vi "Main.vi"(11 "Module Admin":refnum<class "Delacor_lib_QMH_Module Admin.lvclass">) -> ()   [LabVIEW 2020, in "Numpad.lvlib"]
doc: "This template is based off of the Queued Message Handler design pattern and the Queued Message Handler project template that ships with LabVIEW.\n\nThe main difference is that the queue is private to this module and communication between modules is performed via Broadcast and Request events.\n\nRequest events are wrapped in public API methods and are handled in the Event Handling Loop (EHL) of this VI. Any module can register for Broadcast events sent by this module. The EHL generates messages based on user interface actions.\n\nThe Message Handling Loop (MHL) processes messages generated by the EHL, or by other messages. The messages are string values, so new messages can be added easily to the Message Cases case structure in the MHL. Each message cluster can also provide an optional value for Message Data, which is a variant that can be converted to whatever message-specific data is required.\n_____\nBased on Delacor QMH Project Template 5.0.0.82."
uses:
  Numpad.lvlib
  <vilib>/Delacor/Delacor QMH/Libraries/Module Admin_class/Delacor_lib_QMH_Module Admin.lvclass
  Module Data--cluster.ctl
  Stop Argument--cluster.ctl
  <vilib>/Delacor/Delacor QMH/Libraries/Message Queue_class/Delacor_lib_QMH_Message Queue.lvclass/Delacor_lib_QMH_Message Queue.ctl
  <vilib>/Delacor/Delacor QMH/Libraries/Module Admin_class/Delacor_lib_QMH_Module Admin.lvclass/Delacor_lib_QMH_Module Admin.ctl
  Insertar en Subpanel Argument--cluster.ctl
  <vilib>/Utility/miscctls.llb/LVPointTypeDef.ctl
  <vilib>/Delacor/Delacor QMH/Libraries/Message Queue_class/Delacor_lib_QMH_Enqueue Message (Single).vi
  <vilib>/Delacor/Delacor QMH/Libraries/Module Admin_class/Delacor_lib_QMH_Get External Launch.vi
  <vilib>/Utility/error.llb/Error Cluster From Error Code.vi
  <vilib>/ErrorRing/Error Ring.xnode
  <vilib>/Delacor/Delacor QMH/Libraries/Message Queue_class/Delacor_lib_QMH_Message Queue.lvclass
panel:
  out "number":i32
  in  "ok":bool
  in  "0":bool
  in  "del":bool
  in  "9":bool
  in  "8":bool
  in  "7":bool
  in  "6":bool
  in  "5":bool
  in  "4":bool
  in  "3":bool
  in  "2":bool
  in  "1":bool
  out "error out":errorcluster
  out "Status":string
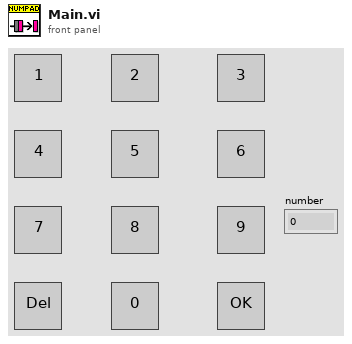
[diagram p1: front panel]
types:
  T1 = typedef "Numpad.lvlib/Request Events--cluster.ctl" = cluster{"Stop Module":refnum<user-event>, "Show Panel":refnum<user-event>, "Hide Panel":refnum<user-event>, "Get Module Execution Status":refnum<user-event>, "Show Diagram":refnum<user-event>, "Insertar en Subpanel":refnum<user-event>}
  T2 = typedef "Numpad.lvlib/Module Data--cluster.ctl" = cluster{"Status":string}
  T3 = enum32{"invalid lock state", "Not Locked", "Locked (No Password)", "Password-protected"}
  T4 = typedef "Numpad.lvlib/Stop Argument--cluster.ctl" = cluster{"Origin":string, "Exit via Stop Module Req?":bool, "Wait for Module to stop?":bool}
  T5 = typedef "Numpad.lvlib/Insertar en Subpanel Argument--cluster.ctl" = cluster{"Subpanel Ref":refnum<vi>}
  T6 = typedef "LVPointTypeDef.ctl" = cluster{"Horizontal":i16, "Vertical":i16}
  T7 = enum32{"Invalid", "Standard", "Closed", "Hidden", "Minimized", "Maximized"}
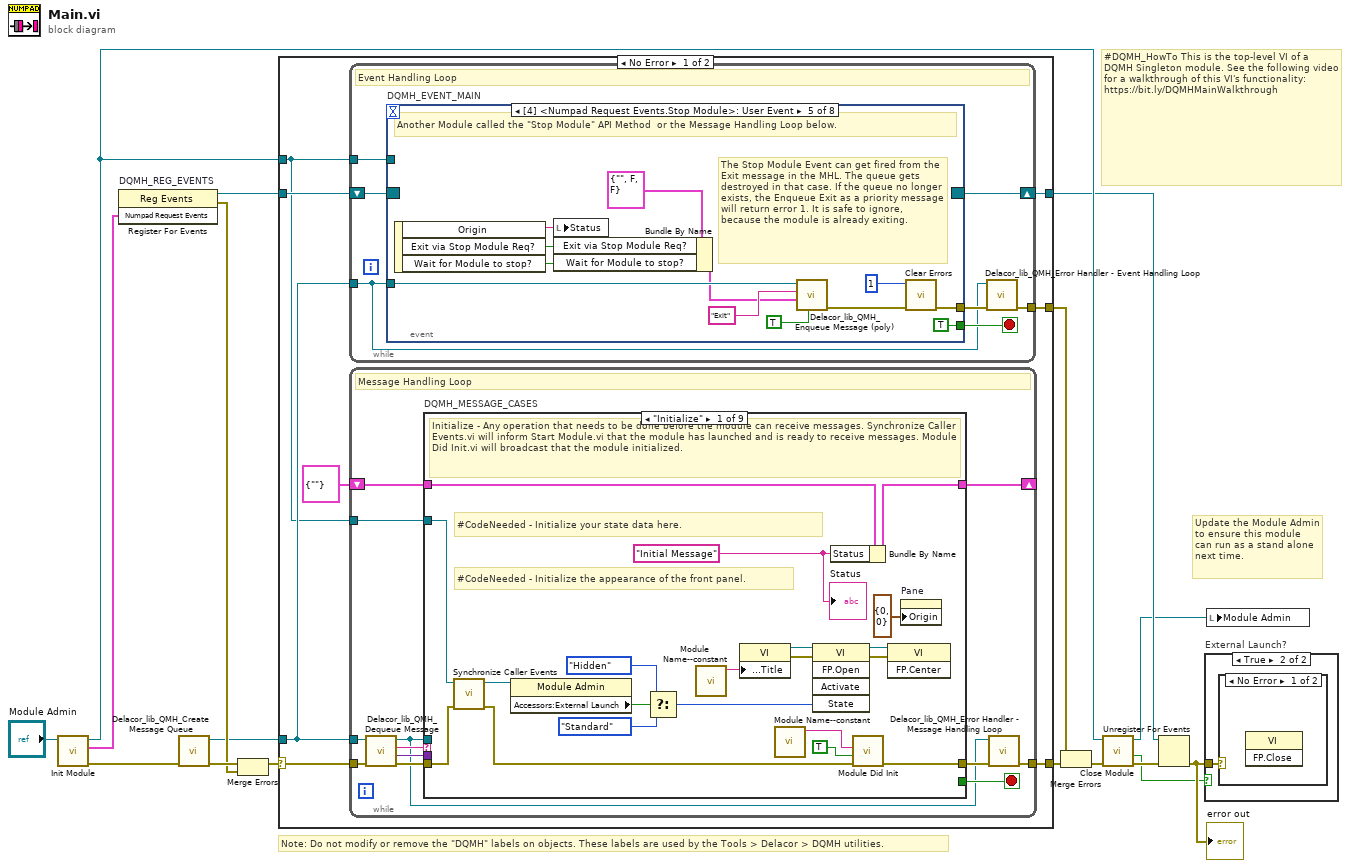
[diagram p0: block diagram]
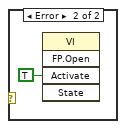
[diagram p3: hidden frame]
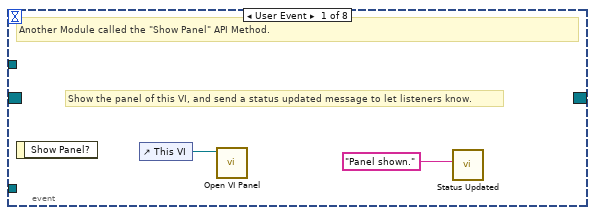
[diagram p4: hidden frame]
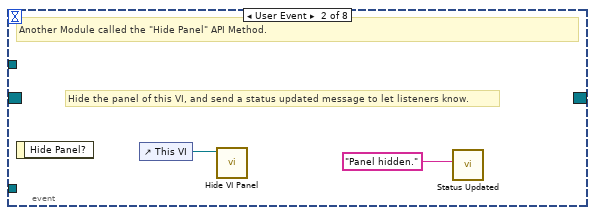
[diagram p5: hidden frame]
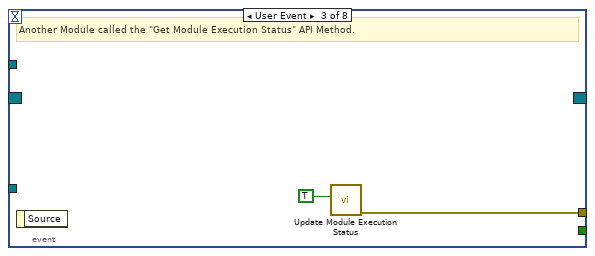
[diagram p6: hidden frame]
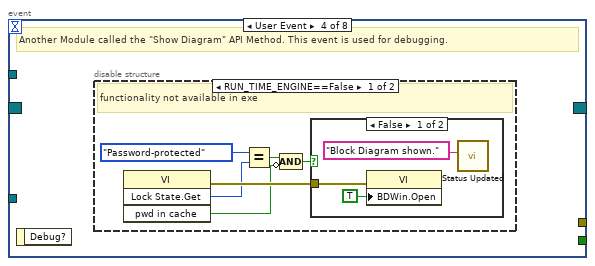
[diagram p7: hidden frame]
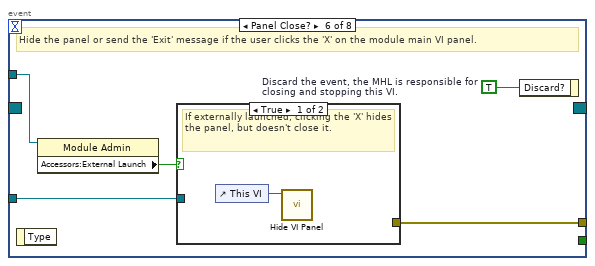
[diagram p10: hidden frame]
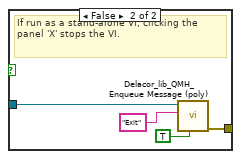
[diagram p11: hidden frame]
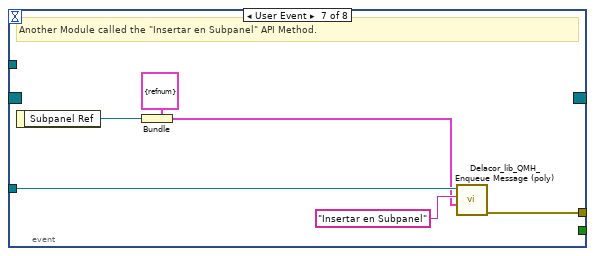
[diagram p12: hidden frame]
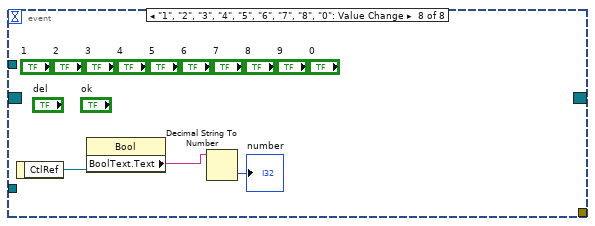
[diagram p13: hidden frame]
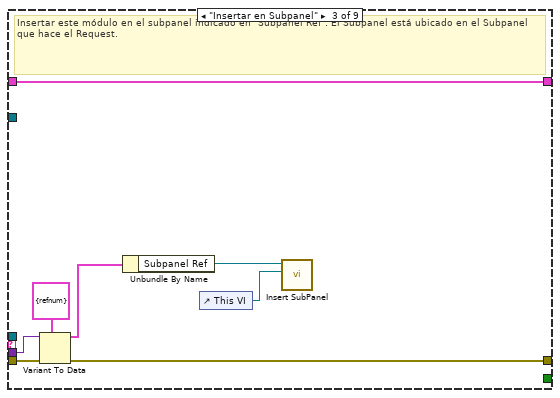
[diagram p15: hidden frame]
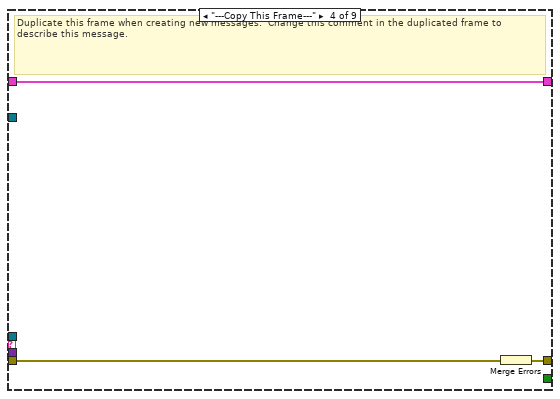
[diagram p16: hidden frame]
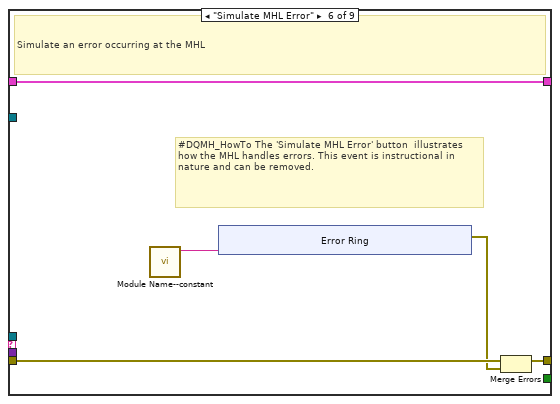
[diagram p18: hidden frame]
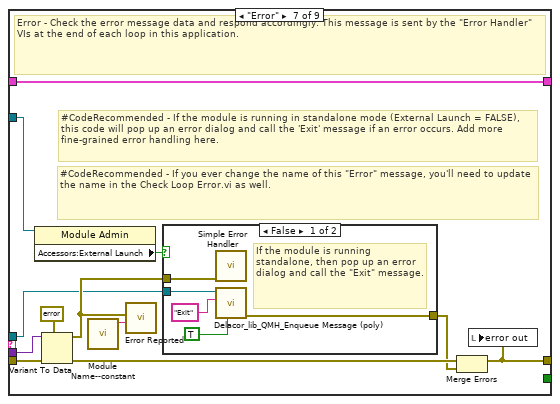
[diagram p19: hidden frame]
diagram:
  # "#DQMH_HowTo This is the top-level VI of a DQMH Singleton module. See the following video for a walkthrough of this VI's functionality: https://bit.ly/DQMHMainWalkthrough"
  # "Note: Do not modify or remove the \"DQMH\" labels on objects. These labels are used by the Tools > Delacor > DQMH utilities."
  # "Update the Module Admin to ensure this module can run as a stand alone next time."
  n1 = call "Init Module.vi"("Singleton Module Admin in"="Module Admin") -> ("error out"=w16:errorcluster, "Numpad Request Events"=w5:T1, "Singleton Module Admin out"=w8:refnum<class "Delacor_lib_QMH_Module Admin.lvclass">)  [unwired: 8 in]
  n2 = register-events "DQMH_REG_EVENTS"(w5) -> (reference out=w6:refnum<event-registration>, error out=w9:errorcluster)  [unwired: 2 in]
  n3 = call <vilib>:"Delacor_lib_QMH_Create Message Queue.vi"("error in (no error)"=w16) -> ("error out"=w11:errorcluster, "Message Queue"=w4:refnum<class "Delacor_lib_QMH_Message Queue.lvclass">)  [unwired: 9 in]
  n4 = Merge Errors(w11, w9) -> (w10:errorcluster)
  n5 = case shown="No Error" w10 {
    selector: w10 -> [w23 w186]
    tunnel: [w25 w185] -> w17
    tunnel: [w22 w191] -> w7
    tunnel: w6 -> [w20 w191]
    tunnel: w4 -> [w19 w184]
    tunnel: [w24 _] -> w14
    tunnel: w8 -> [w18 w187]
    frame No Error {
      n6 = while {
        tunnel: w19 -> [w26]
        shift-right: [w29] -> w22
        shift-left: w20 -> [w30]
        tunnel: [w31] -> w24
        tunnel: w18 -> [w27]
        stop <- w28 stop-if-true
        # "Event Handling Loop"
        n7 = event "DQMH_EVENT_MAIN" shown="[4] <Numpad Request Events.Stop Module>: User Event" {
          selector: w30 -> [_ _ _ _ _ _ _ _]
          dyn-events: [_ _ _ _ _ _ _ _] -> w29
          timeout: _ -> [_ _ _ _ _ _ _ _]
          tunnel: [_ _ _ _ TRUE ("Discard?") _ _ _] -> w28
          tunnel: w26 -> [_ _ _ _ w55 w62 w75 _]
          tunnel: [_ _ w38 _ w58 w64 w70 _] -> w32
          tunnel: w27 -> [_ _ _ _ _ w61 _ _]
          event User Event {
            # "Show the panel of this VI, and send a status updated message to let listeners know."
            # "Another Module called the \"Show Panel\" API Method."
            n8 = event-data() -> ()  [unwired: 1 in, 1 out]
            n9 = control-ref of="This VI"() -> (w34:refnum<vi>)
            n10 = call "Open VI Panel.vi"("VI"=w34) -> ()  [unwired: 10 in, 1 out]
            n11 = call "Status Updated.vi"("Status"="Panel shown." ("format string")) -> ()  [unwired: 10 in, 1 out]
          }
          event User Event {
            # "Hide the panel of this VI, and send a status updated message to let listeners know."
            # "Another Module called the \"Hide Panel\" API Method."
            n12 = event-data() -> ()  [unwired: 1 in, 1 out]
            n13 = control-ref of="This VI"() -> (w36:refnum<vi>)
            n14 = call "Hide VI Panel.vi"("VI"=w36) -> ()  [unwired: 10 in, 1 out]
            n15 = call "Status Updated.vi"("Status"="Panel hidden." ("format string")) -> ()  [unwired: 10 in, 1 out]
          }
          event User Event {
            # "Another Module called the \"Get Module Execution Status\" API Method."
            n16 = event-data() -> ()  [unwired: 1 in, 1 out]
            n17 = call "Update Module Execution Status.vi"("Running?"=TRUE) -> ("error out"=w38:errorcluster)  [unwired: 10 in]
          }
          event User Event {
            # "Another Module called the \"Show Diagram\" API Method. This event is used for debugging."
            n18 = event-data() -> ()  [unwired: 1 in, 1 out]
            n19 = disable-structure shown="RUN_TIME_ENGINE==False" {
              frame condition #0 (active) {
                # "functionality not available in exe"
                n20 = invoke class="VI" method="Lock State.Get"() -> (error out=w44:errorcluster, "Get Lock State"=w43:T3, "pwd in cache"=w40:bool)  [unwired: 4 in, 1 out]
                n21 = Equal?(x=T3."Password-protected", y=w43) -> (x = y?=w41:bool)
                n22 = Compound Arithmetic op=AND(w41, invert w40) -> (w39:bool)
                n23 = case shown="False" w39 {
                  tunnel: w44 -> [w47 _]
                  frame False {
                    n24 = property class="VI"(error in=w47, "BDWin.Open"=TRUE ("Block Diagram Window:Open")) -> ()  [unwired: 1 in, 2 out]
                    n25 = call "Status Updated.vi"("Status"="Block Diagram shown." ("format string")) -> ()  [unwired: 10 in, 1 out]
                  }
                  frame True {
                    # "Password-protected VI, and the password is not in the cache. Do not show the diagram."
                  }
                }
              }
              frame condition #1 {
              }
            }
          }
          event User Event {
            # "The Stop Module Event can get fired from the Exit message in the MHL. The queue gets destroyed in that case. If the queue no longer exists, the Enqueue Exit as a priority message will return error 1. It is safe to ignore, because the module is already exiting."
            # "Another Module called the \"Stop Module\" API Method  or the Message Handling Loop below."
            n26 = event-data() -> ("Origin"=w54:string, "Exit via Stop Module Req?"=w50:bool, "Wait for Module to stop?"=w49:bool)  [unwired: 1 in]
            n27 = local write "Status"(w54) -> ()
            n28 = Bundle By Name(cluster=T4 {"Origin"="", "Exit via Stop Module Req?"=FALSE, "Wait for Module to stop?"=FALSE} ("Stop Argument"), "Exit via Stop Module Req?"=w50, "Wait for Module to stop?"=w49) -> (w48:T4)
            n29 = call-poly <vilib>:"Delacor_lib_QMH_Enqueue Message (poly).vi"("Priority Message? (F)"=TRUE, "Message Data"=w48, "Message"="Exit", "Message Queue in"=w55) -> ("error out"=w59:errorcluster)  [unwired: 6 in, 1 out]
            n30 = call <vilib>:"Clear Errors.vi"("error in (no error)"=w59, "specific error code to clear (0: all)"=1) -> ("error out"=w58:errorcluster)  [unwired: 4 in, 1 out]
          }
          event Panel Close? {
            w63 = TRUE  # Discard the event, the MHL is responsible for closing and stopping this VI.
            # "Hide the panel or send the 'Exit' message if the user clicks the 'X' on the module main VI panel."
            n31 = event-data() -> ()  [unwired: 1 in, 1 out]
            n32 = property class="Module Admin"(reference=w61) -> ("Accessors:External Launch"=w60:bool)  [unwired: 1 in, 2 out]
            n33 = case shown="True" w60 {
              tunnel: w62 -> [_ w68]
              tunnel: [_ w69] -> w64
              frame True {
                # "If externally launched, clicking the 'X' hides the panel, but doesn't close it."
                n34 = control-ref of="This VI"() -> (w65:refnum<vi>)
                n35 = call "Hide VI Panel.vi"("VI"=w65) -> ()  [unwired: 10 in, 1 out]
              }
              frame False {
                # "If run as a stand-alone VI, clicking the panel 'X' stops the VI."
                n36 = call-poly <vilib>:"Delacor_lib_QMH_Enqueue Message (poly).vi"("Priority Message? (F)"=TRUE, "Message"="Exit", "Message Queue in"=w68) -> ("error out"=w69:errorcluster)  [unwired: 7 in, 1 out]
              }
            }
            n37 = event-data("Discard?"=w63) -> ()  [unwired: 1 in, 1 out]
          }
          event User Event {
            # "Another Module called the \"Insertar en Subpanel\" API Method."
            n38 = event-data() -> ("Subpanel Ref"=w71:refnum<vi>)  [unwired: 1 in]
            n39 = Bundle(cluster=T5 {"Subpanel Ref"=refnum} ("Insertar en Subpanel Argument"), "Subpanel Ref"=w71) -> (w72:T5)
            n40 = call-poly <vilib>:"Delacor_lib_QMH_Enqueue Message (poly).vi"("Message Data"=w72, "Message"="Insertar en Subpanel", "Message Queue in"=w75) -> ("error out"=w70:errorcluster)  [unwired: 7 in, 1 out]
          }
          event "1", "2", "3", "4", "5", "6", "7", "8", "0": Value Change {
            n41 = event-data() -> ("CtlRef"=w78:refnum<vi>)  [unwired: 1 in]
            n42 = property class="Bool"(reference=w78) -> ("BoolText.Text"=w77:string)  [unwired: 1 in, 2 out]
            n43 = Decimal String To Number(string=w77) -> (number=→"number":i32)  [unwired: 2 in, 1 out]
          }
        }
        n44 = call-dynamic "Delacor_lib_QMH_Error Handler - Event Handling Loop.vi"("error in (no error)"=w32, "Message Queue in"=w26) -> ("dup error in"=w31:errorcluster)  [unwired: 8 in, 1 out]
      }
      n45 = while {
        tunnel: w19 -> [w81]
        shift-right: [w85] -> _
        shift-left: T2 {"Status"=""} ("Data Cluster") -> [w86]
        tunnel: w23 -> [w89]
        tunnel: [w87] -> w25
        tunnel: w18 -> [w79]
        stop <- w84 stop-if-true
        # "Message Handling Loop"
        n46 = call-dynamic "Delacor_lib_QMH_Dequeue Message.vi"("error in (no error)"=w89, "Message Queue in"=w81) -> ("error out"=w88:errorcluster, "Message Data"=w82:variant, "Message"=w83:string, "Message Queue out"=w80:refnum<class "Delacor_lib_QMH_Message Queue.lvclass">)  [unwired: 6 in]
        n47 = case "DQMH_MESSAGE_CASES" shown="\"Initialize\"" w83 {
          selector: w83 -> [_ _ _ _ _ _ _ _ w171]
          tunnel: w80 -> [_ _ _ _ _ _ w141 w163 _]
          tunnel: w88 -> [w108 w112 w120 w123 w125 w130 w148 w169 w173]
          tunnel: [w106 w112 w118 w122 w125 w129 w144 w166 w174] -> w90
          tunnel: w86 -> [w97 w111 w119 w121 w124 w127 w143 w162 w172]
          tunnel: [w96 w111 w119 w121 w124 w127 w143 w162 w172] -> w85
          tunnel: [_ _ _ _ _ _ _ w161 _] -> w84
          tunnel: w82 -> [_ _ w117 _ _ _ w142 w160 _]
          tunnel: w79 -> [w98 _ _ _ _ _ w140 w155 _]
          frame "Initialize" {
            w91 = "Initial Message" ("Initial Message")
            # "#CodeNeeded - Initialize the appearance of the front panel."
            # "#CodeNeeded - Initialize your state data here."
            # "Initialize - Any operation that needs to be done before the module can receive messages. Synchronize Caller Events.vi will inform Start Module.vi that the module has launched and is ready to receive messages. Module Did Init.vi will broadcast that the module initialized."
            n48 = call "Synchronize Caller Events.vi"("error in (no error)"=w108, "Singleton Module Admin in"=w98) -> ("error out"=w107:errorcluster, "Singleton Module Admin out"=w93:refnum<class "Delacor_lib_QMH_Module Admin.lvclass">)  [unwired: 8 in]
            n49 = property class="Module Admin"(reference=w93) -> ("Accessors:External Launch"=w102:bool)  [unwired: 1 in, 2 out]
            n50 = Select(t=T7."Hidden" ("State"), s=w102, f=T7."Standard" ("State")) -> (s? t:f=w99:T7)
            n51 = call "Module Name--constant.vi"() -> ("Module Name"=w105:string)  [unwired: 11 in]
            n52 = property class="VI"("Front Panel.Title"=w105) -> (reference out=w104:refnum<vi>, error out=w110:errorcluster)  [unwired: 2 in]
            n53 = call "Module Name--constant.vi"() -> ("Module Name"=w94:string)  [unwired: 11 in]
            n54 = invoke class="VI" method="FP.Open"(reference=w104, error in=w110, "State"=w99) -> (reference out=w103:refnum<vi>, error out=w109:errorcluster)  [unwired: 2 in, 3 out]
            n55 = Bundle By Name(cluster=w97, "Status"=w91) -> (w96:T2)
            n56 = call "Module Did Init.vi"("error in (no error)"=w107, "Initialized?"=TRUE, "Origin"=w94) -> ("error out"=w106:errorcluster)  [unwired: 8 in]
            n57 = invoke class="VI" method="FP.Center"(reference=w103, error in=w109) -> ()  [unwired: 1 in, 3 out]
            n58 = property on="Pane" class="Pane"("Origin"=T6 {"Horizontal"=0, "Vertical"=0}) -> ()  [unwired: 2 in, 2 out]
            "Status" <- w91
          }
          frame "--- Module Specific ---" {
            # "Separator -- The following cases handle messages specific to this Module."
          }
          frame "Insertar en Subpanel" {
            # "Insertar este módulo en el subpanel indicado en \"Subpanel Ref\". El Subpanel está ubicado en el Subpanel que hace el Request."
            n59 = Variant To Data(error in=w120, type=T5 {"Subpanel Ref"=refnum} ("Insertar en Subpanel Argument"), Variant=w117) -> (data=w115:T5, error out=w118:errorcluster)
            n60 = Unbundle By Name(w115) -> ("Subpanel Ref"=w114:refnum<vi>)
            n61 = control-ref of="This VI"() -> (w113:refnum<vi>)
            n62 = call "Insert SubPanel.vi"("VI Ref"=w113, "Subpanel Ref"=w114) -> ()  [unwired: 9 in, 1 out]
          }
          frame "---Copy This Frame---" {
            # "Duplicate this frame when creating new messages.  Change this comment in the duplicated frame to describe this message."
            n63 = Merge Errors(w123) -> (w122:errorcluster)
          }
          frame "--- Exit and Error Handling---" {
            # "Separator - The following cases handle errors and exit messages."
          }
          frame "Simulate MHL Error" {
            # "#DQMH_HowTo The 'Simulate MHL Error' button  illustrates how the MHL handles errors. This event is instructional in nature and can be removed."
            # "Simulate an error occurring at the MHL"
            n64 = call "Module Name--constant.vi"() -> ("Module Name"=w126:string)  [unwired: 11 in]
            n65 = xnode "Error Ring"("parameter 0"=w126) -> ("error out"=w128:errorcluster)
            n66 = Merge Errors(w130, w128) -> (w129:errorcluster)
          }
          frame "Error" {
            # "#CodeRecommended - If you ever change the name of this \"Error\" message, you'll need to update the name in the Check Loop Error.vi as well."
            # "#CodeRecommended - If the module is running in standalone mode (External Launch = FALSE), this code will pop up an error dialog and call the 'Exit' message if an error occurs. Add more fine-grained error handling here."
            # "Error - Check the error message data and respond accordingly. This message is sent by the \"Error Handler\" VIs at the end of each loop in this application."
            n67 = property class="Module Admin"(reference=w140) -> ("Accessors:External Launch"=w139:bool)  [unwired: 1 in, 2 out]
            n68 = Variant To Data(error in=w148, type=errorcluster {"status"=FALSE, "code"=0, "source"=""} ("error constant"), Variant=w142) -> (data=w149:errorcluster, error out=w146:errorcluster)
            n69 = call "Module Name--constant.vi"() -> ("Module Name"=w138:string)  [unwired: 11 in]
            n70 = call "Error Reported.vi"("Additional Information"=w138, "Error"=w149) -> ()  [unwired: 9 in, 1 out]
            n71 = case shown="False" w139 {
              tunnel: [w154 _] -> w145
              tunnel: w141 -> [w152 _]
              tunnel: w149 -> [w153 _]
              frame False {
                # "If the module is running standalone, then pop up an error dialog and call the \"Exit\" message."
                n72 = call <vilib>:"Simple Error Handler.vi"("error in (no error)"=w153) -> ()  [unwired: 4 in, 5 out]
                n73 = call-poly <vilib>:"Delacor_lib_QMH_Enqueue Message (poly).vi"("Priority Message? (F)"=TRUE, "Message"="Exit", "Message Queue in"=w152) -> ("error out"=w154:errorcluster)  [unwired: 7 in, 1 out]
              }
              frame True {
                # "If the module was launched externally, calling the Error Reported broadcast VI is the only action performed by the \"Error\" message. The module's caller can then process the error appropriately."
              }
            }
            n74 = Merge Errors(w146, w145) -> (w144:errorcluster)
            n75 = local write "error out"(w144) -> ()
          }
          frame "Exit" {
            w159 = 91  # 91: not all Exit messages will have an argument
            w161 = TRUE  # Stop the VI
            # "Release the message queue reference"
            # "#CodeNeeded - Add any required cleanup code here"
            # "Exit - Exit the application."
            n76 = Variant To Data(error in=w169, type=T4 {"Origin"="", "Exit via Stop Module Req?"=FALSE, "Wait for Module to stop?"=FALSE} ("Stop Argument"), Variant=w160) -> (data=w157:T4, error out=w165:errorcluster)
            n77 = call <vilib>:"Clear Errors.vi"("error in (no error)"=w165, "specific error code to clear (0: all)"=w159) -> ("error out"=w168:errorcluster)  [unwired: 4 in, 1 out]
            n78 = control-ref of="This VI"() -> (w156:refnum<vi>)
            n79 = call-dynamic "Delacor_lib_QMH_Release Message Queue.vi"("error in (no error)"=w168, "Message Queue"=w163) -> ("error out"=w167:errorcluster)  [unwired: 9 in]
            n80 = call "Handle Exit.vi"("Stop Argument"=w157, "Admin in"=w155, "VI reference"=w156) -> ("error out"=w164:errorcluster)  [unwired: 7 in, 1 out]
            n81 = Merge Errors(w167, w164) -> (w166:errorcluster)
          }
          frame Default {
            # "'Default' case only runs if there is a message that isn't defined in any of the other cases.  Output a programming error."
            n82 = call "Module Name--constant.vi"() -> ("Module Name"=w170:string)  [unwired: 11 in]
            n83 = xnode "Error Ring"("parameter 0"=w171, "parameter 1"=w170) -> ("error out"=w175:errorcluster)
            n84 = Merge Errors(w173, w175) -> (w174:errorcluster)
          }
        }
        n85 = call-dynamic "Delacor_lib_QMH_Error Handler - Message Handling Loop.vi"("error in (no error)"=w90, "Message Queue in"=w80) -> ("dup error in"=w87:errorcluster)  [unwired: 8 in, 1 out]
      }
    }
    frame Error {
      # "Synchronize Caller Events.vi will inform Start Module.vi that the module has launched and will let the code calling Start Module.vi register for broadcasts and would permit the caller receive the broadcast that an error occurred at launch time."
      n86 = call-dynamic "Delacor_lib_QMH_Release Message Queue.vi"("error in (no error)"=w186, "Message Queue"=w184) -> ("error out"=w185:errorcluster)  [unwired: 9 in]
      n87 = call "Synchronize Caller Events.vi"("Singleton Module Admin in"=w187) -> ("error out"=w192:errorcluster)  [unwired: 9 in, 1 out]
      n88 = call "Module Name--constant.vi"() -> ("Module Name"=w190:string)  [unwired: 11 in]
      n89 = Format Into String(format string="An error occurred during initialization. %s is no longer running.", w190) -> (resulting string=w188:string)  [unwired: 2 in, 1 out]
      n90 = Merge Errors(w185, w192) -> (w193:errorcluster)
      n91 = call "Error Reported.vi"("Additional Information"=w188, "Error"=w193) -> ()  [unwired: 9 in, 1 out]
    }
  }
  n92 = Merge Errors(w14, w17) -> (w13:errorcluster)
  n93 = call "Close Module.vi"("error in (no error)"=w13, "Module Admin in"=w8) -> ("error out"=w15:errorcluster, "External Launch"=w1:bool, "Module Admin out"=w2:refnum<class "Delacor_lib_QMH_Module Admin.lvclass">)  [unwired: 7 in]
  n94 = Unregister For Events(event registration refnum=w7, error in=w15) -> (error out=w12:errorcluster)
  "error out" <- w12
  n95 = case "External Launch?" shown="True" w1 {
    tunnel: w12 -> [_ w194]
    frame False {
    }
    frame True {
      n96 = case shown="No Error" w194 {
        frame No Error {
          n97 = invoke class="VI" method="FP.Close"() -> ()  [unwired: 3 in, 3 out]
        }
        frame Error {
          n98 = invoke class="VI" method="FP.Open"("Activate"=TRUE ("Activate?")) -> ()  [unwired: 4 in, 5 out]
        }
      }
    }
  }
  n99 = local write "Module Admin"(w2) -> ()
